vi "FRCts20_Backend_GenTeamEntries.vi"() -> ()   [LabVIEW 2014, in "FRCts20_Backend_TestCode.lvlib"]
uses:
  FRCts20_Backend_TestCode.lvlib
  FRCts20_Backend_WebMethods.lvlib
  FRCts20_Backend_IssueDfn.ctl
  FRCts20_Backend_Controls.lvlib
  FRCts20_Backend_TeamDfn.ctl
  FRCts20_Backend_Team_Info.ctl
  FRCts20_Backend_Note.ctl
  FRCts20_Backend_Note_list.ctl
  FRCts20_Backend_request_info.ctl
  FRCts20_Backend_IssueTeamList.ctl
panel:
  out "Array":string[](array[string])
  in  "NumTeams":i32
  in  "Team":T1
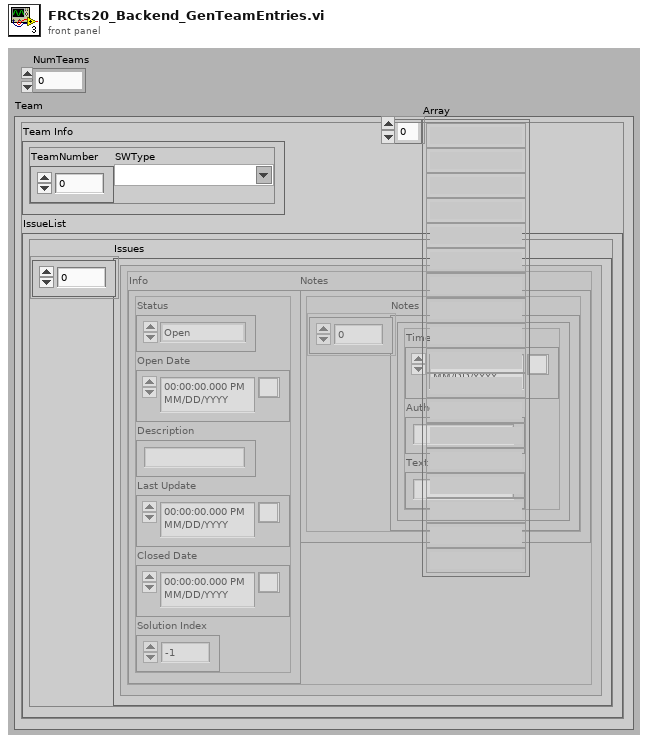
[diagram p1: front panel]
types:
  T1 = typedef "FRCts20_Backend_Controls.lvlib/FRCts20_Backend_TeamDfn.ctl" = cluster{"Team Info":T2, "IssueList":T3}
  T2 = typedef "FRCts20_Backend_Controls.lvlib/FRCts20_Backend_Team_Info.ctl" = cluster{"TeamNumber":u16, "SWType":string}
  T3 = typedef "FRCts20_Backend_Controls.lvlib/FRCts20_Backend_IssueTeamList.ctl" = cluster{"Issues":T4[]}
  T4 = typedef "FRCts20_Backend_Controls.lvlib/FRCts20_Backend_IssueDfn.ctl" = cluster{"Notes":T5, "Info":T7}
  T5 = typedef "FRCts20_Backend_Controls.lvlib/FRCts20_Backend_Note_list.ctl" = cluster{"Notes":T6[]}
  T6 = typedef "FRCts20_Backend_Controls.lvlib/FRCts20_Backend_Note.ctl" = cluster{"Time Entered":timestamp, "Author":string, "Text":string}
  T7 = typedef "FRCts20_Backend_Controls.lvlib/FRCts20_Backend_request_info.ctl" = cluster{"Status":enum16{"Open", "In Work", "Closed"}, "Open Date":timestamp, "Description":string, "Last Update":timestamp, "Closed Date":timestamp, "Solution Index":i32}
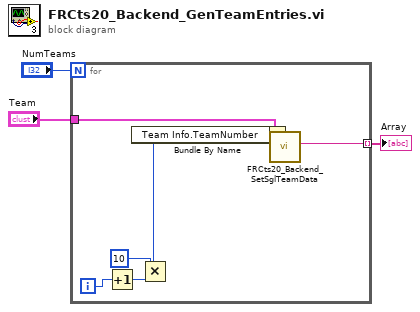
[diagram p0: block diagram]
diagram:
  n1 = for {
    N: "NumTeams" -> [_]
    tunnel: "Team" -> [w10]
    tunnel: [w4] -> w1 mode=indexing
    i -> [w9]
    n2 = Increment(x=w9) -> (x+1=w8:i32)
    n3 = Multiply(x=10, y=w8) -> (x*y=w6:i32)
    n4 = Bundle By Name(cluster=w10, "Team Info.TeamNumber"=w6) -> (w5:T1)
    n5 = call "FRCts20_Backend_SetSglTeamData.vi"("Team"=w5) -> ("Status?"=w4:string)  [unwired: 9 in, 1 out]
  }
  "Array" <- w1
